vi "Get Analog Replay Data Options.vi"(8 "error in (no error)":errorcluster, 11 "NodeID":u64) -> (0 "error out":errorcluster, 2 "Analog Replay Data Options":T1={"Selected File"=path "", "Group"="", "Channel"="", "DataPlugin"="", "ReverseData"=FALSE, "FPGA memory size"=enum."16,384", "CycleAngle?"=enum."Crank angle", "Data Selection Method"=enum."Manual", "File start offset"=1, "Samples"=1, "Missing teeth location (degrees)"=1.0} {"Missing teeth location (degrees)" min=0.0; "Samples" min=1; "File start offset" min=0}, 3 "NodeID":u64)   [LabVIEW 2015, in "Engine Simulation Toolkit Scripting API.lvlib"]
uses:
  Engine Simulation Toolkit Scripting API.lvlib
  Analog Replay Data Options.ctl
  System Explorer/FPGA Mem Size.ctl
  System Explorer/Position Reference.ctl
  System Explorer/Data Replay Data Selection Method.ctl
  System Explorer/Engine Simulation Toolkit System Explorer.lvlib
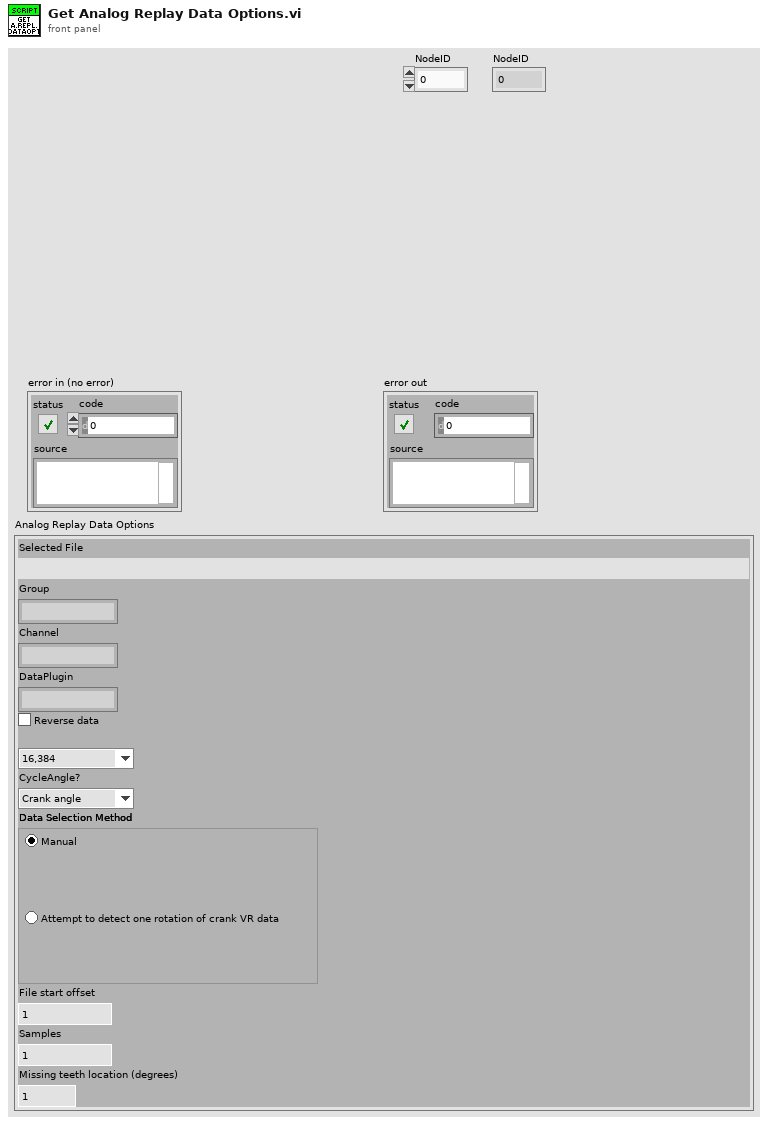
[diagram p1: front panel]
types:
  T1 = typedef "Engine Simulation Toolkit Scripting API.lvlib/Analog Replay Data Options.ctl" = cluster{"Selected File":path, "Group":string, "Channel":string, "DataPlugin":string, "ReverseData":bool, "FPGA memory size":T2, "CycleAngle?":T3, "Data Selection Method":T4, "File start offset":i32, "Samples":i32, "Missing teeth location (degrees)":dbl}
  T2 = typedef "Engine Simulation Toolkit System Explorer.lvlib/FPGA Mem Size.ctl" = enum16{"65,536", "32,768", "16,384", "8,192", "4,096", "2,048", "1,024"}
  T3 = typedef "Engine Simulation Toolkit System Explorer.lvlib/Position Reference.ctl" = enum16{"Crank angle", "Cycle angle"}
  T4 = typedef "Engine Simulation Toolkit System Explorer.lvlib/Data Replay Data Selection Method.ctl" = enum32{"Manual", "AutoVRCrank"}
  T5 = typedef "Engine Simulation Toolkit System Explorer.lvlib/File Load Dialog.ctl" = cluster{"File":path, "Group":string, "Channel":string, "DataPlugin":string, "MissingTeeth":dbl, "ErrState":string, "File Selected":bool, "Data Selection Method":T4, "Offset":i32, "Length":i32, "DataPlugins Info":T6[], "Controls":refnum<vi>[], "File Ref":refnum<k20>, "Groups":string[], "Channels":string[], "Groups Refs":refnum<k20>[], "Channel Refs":refnum<k20>[], "Cancelled":bool, "Position reference":T3, "FPGA memory size":T2, "GroupRef":refnum<k20>, "ChanRef":refnum<k20>, "Data":dbl[], "ReverseData":bool, "DispTwoRotations":bool, "cycle range":u16}
  T6 = typedef "usiPluginInformation.ctl" = cluster{"name":string, "version":string, "type":string, "read-only?":bool, "extensions":string[]}
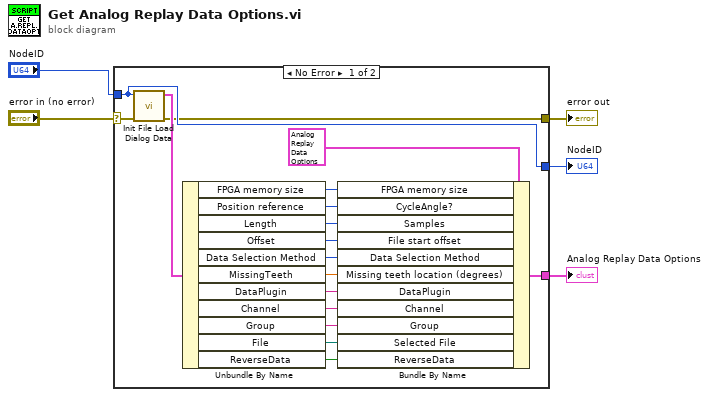
[diagram p0: block diagram]
diagram:
  n1 = case shown="No Error" "error in (no error)" {
    selector: "error in (no error)" -> [w8 w24]
    tunnel: "NodeID" -> [w9 w23]
    tunnel: [w7 w24] -> w3
    tunnel: [w9 w23] -> w2
    tunnel: [w6 _] -> w1
    frame No Error {
      n2 = call "Init File Load Dialog Data.vi"("error in (no error)"=w8, "Node Ptr"=w9) -> ("error out"=w7:errorcluster, "FileDialog"=w22:T5)  [unwired: 8 in]
      n3 = Unbundle By Name(w22) -> ("FPGA memory size"=w20:T2, "Position reference"=w19:T3, "Length"=w18:i32, "Offset"=w17:i32, "Data Selection Method"=w16:T4, "MissingTeeth"=w15:dbl, "DataPlugin"=w14:string, "Channel"=w13:string, "Group"=w12:string, "File"=w11:path, "ReverseData"=w10:bool)
      n4 = Bundle By Name(cluster=T1 {"Selected File"=path "", "Group"="", "Channel"="", "DataPlugin"="", "ReverseData"=FALSE, "FPGA memory size"=enum."16,384", "CycleAngle?"=enum."Crank angle", "Data Selection Method"=enum."Manual", "File start offset"=1, "Samples"=1, "Missing teeth location (degrees)"=1.0} ("Analog Replay Data Options"), "FPGA memory size"=w20, "CycleAngle?"=w19, "Samples"=w18, "File start offset"=w17, "Data Selection Method"=w16, "Missing teeth location (degrees)"=w15, "DataPlugin"=w14, "Channel"=w13, "Group"=w12, "Selected File"=w11, "ReverseData"=w10) -> (w6:T1)
    }
    frame Error {
    }
  }
  "error out" <- w3
  "NodeID" <- w2
  "Analog Replay Data Options" <- w1
